vi "Add View.vi"(8 "error in (no error)":errorcluster, 9 "View Details":T1, 10 "View":string, 11 "GUI Container View Actor in":refnum<class "GUI Container.lvclass">) -> (0 "error out":errorcluster, 3 "GUI Container View Actor out":refnum<class "GUI Container.lvclass">)   [LabVIEW 2023, in "GUI Views.lvlib" / "GUI Container.lvclass"]
doc: "This method is called by the a contained GUI View to allow the GUI Container to store the GUI VIew details"
uses:
  GUI Container.lvclass
  typedefs/View Details.ctl
  <vilib>/ActorFramework/Message Enqueuer/Message Enqueuer.lvclass
  typedefs/View Status.ctl
  typedefs/FP Status.ctl
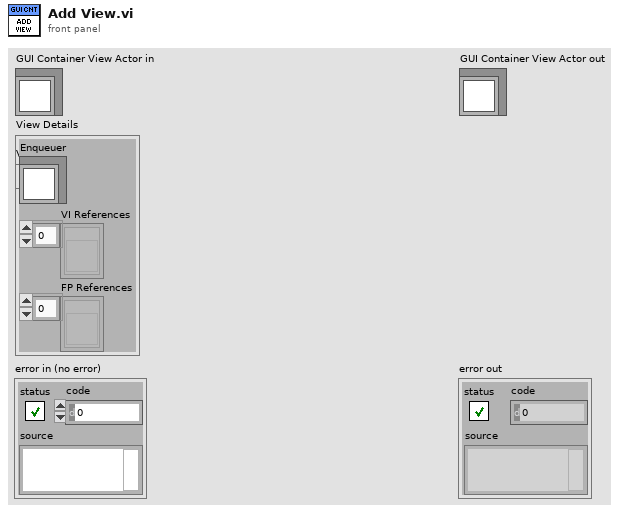
[diagram p1: front panel]
types:
  T1 = typedef "GUI Views.lvlib/GUI Container.lvclass/View Details.ctl" = cluster{"Enqueuer":refnum<class "Message Enqueuer.lvclass">, "VI References":refnum<vi>[], "FP References":refnum<vi>[]}
  T2 = typedef "GUI Views.lvlib/GUI Container.lvclass/View Status.ctl" = cluster{"View Details":T1, "Front Panel Statuses":T3[]}
  T3 = typedef "GUI Views.lvlib/GUI Container.lvclass/FP Status.ctl" = cluster{"FP Open":bool, "Inserted in Subpanel":bool, "Subpanel":string}
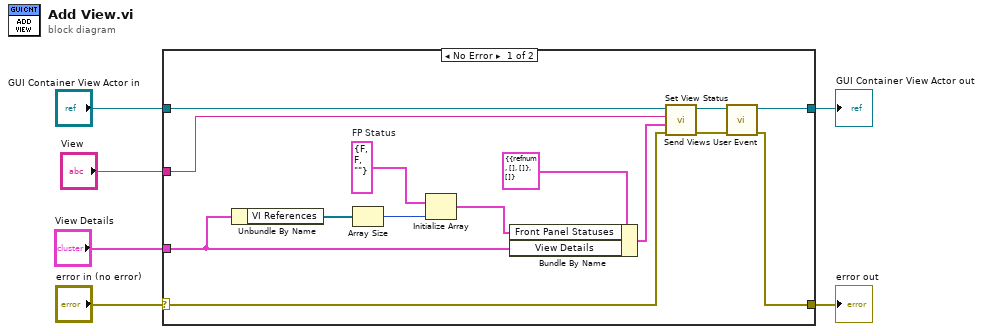
[diagram p0: block diagram]
diagram:
  n1 = case shown="No Error" "error in (no error)" {
    selector: "error in (no error)" -> [w19 w22]
    tunnel: [w14 w22] -> w5
    tunnel: [w16 w21] -> w3
    tunnel: "GUI Container View Actor in" -> [w20 w21]
    tunnel: "View" -> [w18 _]
    tunnel: "View Details" -> [w11 _]
    frame No Error {
      w8 = T3 {"FP Open"=FALSE, "Inserted in Subpanel"=FALSE, "Subpanel"=""}  # FP Status
      n2 = Unbundle By Name(w11) -> ("VI References"=w10:refnum<vi>[])
      n3 = Array Size(array=w10) -> (size(s)=w9:i32)
      n4 = Initialize Array(w8, w9) -> (w7:T3[])
      n5 = Bundle By Name(cluster=T2 {"View Details"={"Enqueuer"=refnum, "VI References"=[], "FP References"=[]}, "Front Panel Statuses"=[]} ("View State"), "Front Panel Statuses"=w7, "View Details"=w11) -> (w12:T2)
      n6 = call "Set View Status.vi"("error in (no error)"=w19, "View Status"=w12, "View"=w18, "GUI Container Actor in"=w20) -> ("error out"=w15:errorcluster, "GUI Container Actor out"=w17:refnum<class "GUI Container.lvclass">)  [unwired: 5 in, 1 out]
      n7 = call "Send Views User Event.vi"("error in (no error)"=w15, "GUI Container Actor in"=w17) -> ("error out"=w14:errorcluster, "GUI Container Actor out"=w16:refnum<class "GUI Container.lvclass">)  [unwired: 8 in]
    }
    frame Error {
    }
  }
  "error out" <- w5
  "GUI Container View Actor out" <- w3
